vi "TwithFPO_DAQmx.vi"() -> ()   [LabVIEW 2019]
doc: "EE 200 Problem Set 7 Problem 25"
uses:
  Downloads/Project 2/Project 2/state.ctl
  <vilib>/DAQmx/read.llb/DAQmx Read (Digital 1D Bool 1Chan 1Samp).vi
  <vilib>/DAQmx/write.llb/DAQmx Write (Digital 1D Bool 1Chan 1Samp).vi
  <vilib>/DAQmx/write.llb/DAQmx Write (Analog DBL 1Chan 1Samp).vi
  <vilib>/DAQmx/read.llb/DAQmx Read (Digital Bool 1Line 1Point).vi
  <vilib>/DAQmx/create/channels.llb/DAQmx Create Channel (DI-Digital Input).vi
  <vilib>/DAQmx/create/channels.llb/DAQmx Create Channel (DO-Digital Output).vi
  <vilib>/DAQmx/create/channels.llb/DAQmx Create Channel (AO-Voltage-Basic).vi
  <vilib>/DAQmx/miscellaneous.llb/DAQmx Fill In Error Info.vi
panel:
  out "Thermostat Signal":u32[](array[colorbox])
  out "Reset":bool
  out "Clock":bool
  out "Present State":T1
  out "Clock Cycle":i32
  out "Sensors":bool[](array[boolean])
  in  "Stop Button":bool
  # "Thermostat"
  # "H\n\nC\n\nB"
  # "Standby \n\n\nCharging\n\n\nCooling\n\n\nHeating"
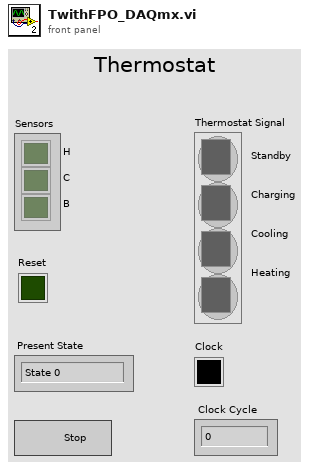
[diagram p1: front panel]
types:
  T1 = typedef "state.ctl" = enum16{"State 0", "State 1", "State 2", "State 3"}
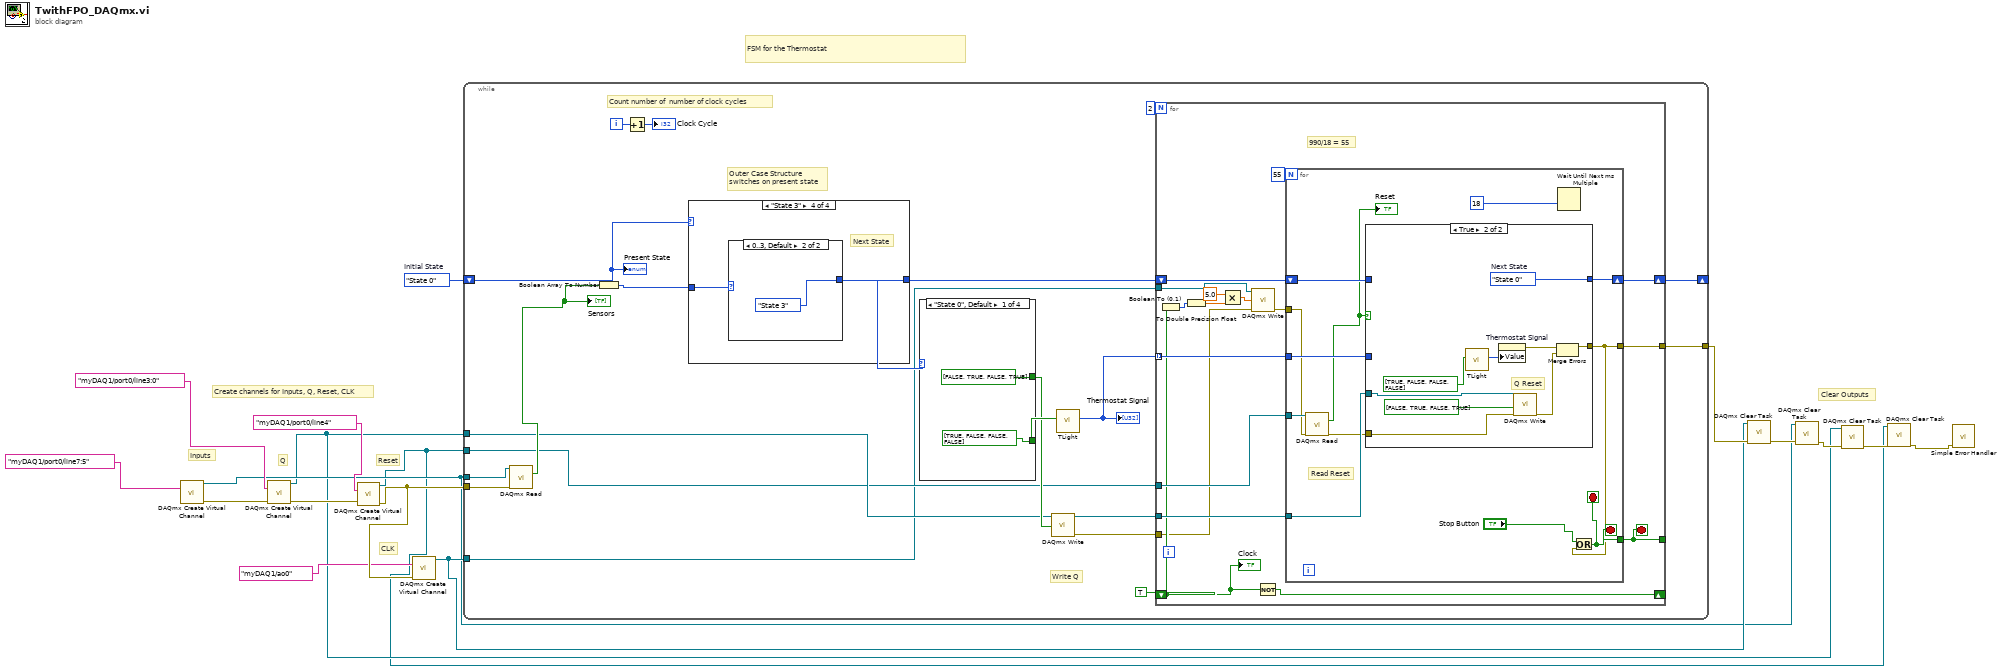
[diagram p0: block diagram]
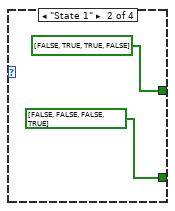
[diagram p2: hidden frame]
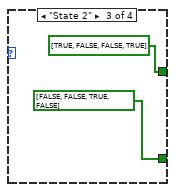
[diagram p3: hidden frame]
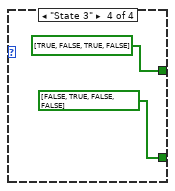
[diagram p4: hidden frame]
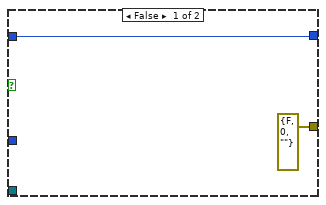
[diagram p5: hidden frame]
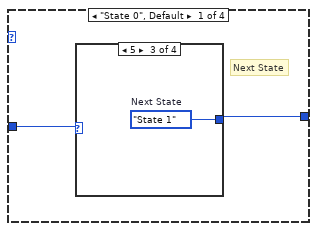
[diagram p6: hidden frame]
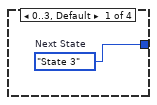
[diagram p7: hidden frame]
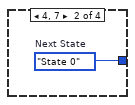
[diagram p8: hidden frame]
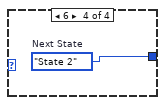
[diagram p9: hidden frame]
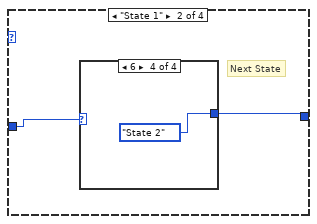
[diagram p10: hidden frame]
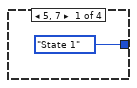
[diagram p11: hidden frame]
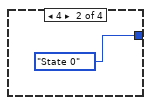
[diagram p12: hidden frame]
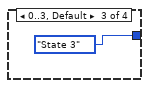
[diagram p13: hidden frame]
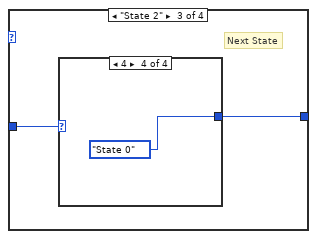
[diagram p14: hidden frame]
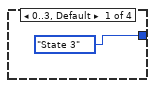
[diagram p15: hidden frame]
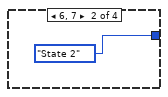
[diagram p16: hidden frame]
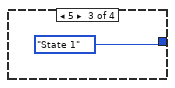
[diagram p17: hidden frame]
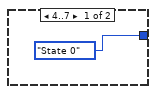
[diagram p18: hidden frame]
diagram:
  w17 = state."State 0"  # Initial State
  # "Clear Outputs"
  # "Create channels for Inputs, Q, Reset, CLK"
  # "CLK"
  # "Reset"
  # "Q"
  # "Inputs"
  # "FSM for the Thermostat"
  n1 = call-poly <vilib>:"DAQmx Create Virtual Channel.vi"("lines"=tag "myDAQ1/port0/line7:5") -> ("task out"=w3:refnum<k21>, "error out"=w16:errorcluster)  [unwired: 13 in]
  n2 = call-poly <vilib>:"DAQmx Create Virtual Channel.vi"("lines"=tag "myDAQ1/port0/line3:0", "error in"=w16) -> ("task out"=w2:refnum<k21>, "error out"=w15:errorcluster)  [unwired: 12 in]
  n3 = call-poly <vilib>:"DAQmx Create Virtual Channel.vi"("lines"=tag "myDAQ1/port0/line4", "error in"=w15) -> ("task out"=w1:refnum<k21>, "error out"=w14:errorcluster)  [unwired: 12 in]
  n4 = call-poly <vilib>:"DAQmx Create Virtual Channel.vi"("physical channels"=tag "myDAQ1/ao0", "error in"=w14) -> ("task out"=w8:refnum<k21>)  [unwired: 12 in, 1 out]
  n5 = while {
    shift-right: [w33] -> _
    shift-left: w17 -> [w36]
    tunnel: [w31] -> w9
    tunnel: w3 -> [w27]
    tunnel: w14 -> [w26]
    tunnel: w2 -> [w22]
    tunnel: w1 -> [w20]
    tunnel: w8 -> [w19]
    i -> [w38]
    stop <- w35 stop-if-true
    # "Write Q"
    # "Count number of  number of clock cycles"
    # "Outer Case Structure \nswitches on present state"
    n6 = call-poly <vilib>:"DAQmx Read.vi"("task/channels in"=w27, "error in"=w26) -> ("data"=w25:bool[])  [unwired: 11 in, 2 out]
    "Sensors" <- w25
    n7 = Boolean Array To Number(Boolean array=w25) -> (number=w28:u32)
    n8 = Increment(x=w38) -> (x+1=→"Clock Cycle":i32)
    n9 = case shown="\"State 3\"" w36 {
      tunnel: [w88 w94 w100 w106] -> w32
      tunnel: w28 -> [w87 w93 w99 w105]
      frame "State 0", Default {
        # "Next State"
        n10 = case shown="5" w87 {
          tunnel: [w89 w90 w91 w92] -> w88
          frame 0..3, Default {
            w89 = state."State 3"  # Next State
          }
          frame 4, 7 {
            w90 = state."State 0"  # Next State
          }
          frame 5 {
            w91 = state."State 1"  # Next State
          }
          frame 6 {
            w92 = state."State 2"  # Next State
          }
        }
      }
      frame "State 1" {
        # "Next State"
        n11 = case shown="6" w93 {
          tunnel: [state."State 1" ("Present State") state."State 0" ("Present State") state."State 3" ("Present State") state."State 2" ("Present State")] -> w94
          frame 5, 7 {
          }
          frame 4 {
          }
          frame 0..3, Default {
          }
          frame 6 {
          }
        }
      }
      frame "State 2" {
        # "Next State"
        n12 = case shown="4" w99 {
          tunnel: [state."State 3" ("Present State") state."State 2" ("Present State") state."State 1" ("Present State") state."State 0" ("Present State")] -> w100
          frame 0..3, Default {
          }
          frame 6, 7 {
          }
          frame 5 {
          }
          frame 4 {
          }
        }
      }
      frame "State 3" {
        # "Next State"
        n13 = case shown="0..3, Default" w105 {
          tunnel: [state."State 0" ("Present State") state."State 3" ("Present State")] -> w106
          frame 4..7 {
          }
          frame 0..3, Default {
          }
        }
      }
    }
    n14 = case shown="\"State 0\", Default" w32 {
      tunnel: [bool[] [TRUE, FALSE, FALSE, FALSE] bool[] [FALSE, FALSE, FALSE, TRUE] bool[] [FALSE, FALSE, TRUE, FALSE] bool[] [FALSE, TRUE, FALSE, FALSE]] -> w24
      tunnel: [bool[] [FALSE, TRUE, FALSE, TRUE] bool[] [FALSE, TRUE, TRUE, FALSE] bool[] [TRUE, FALSE, FALSE, TRUE] bool[] [TRUE, FALSE, TRUE, FALSE]] -> w23
      frame "State 0", Default {
      }
      frame "State 1" {
      }
      frame "State 2" {
      }
      frame "State 3" {
      }
    }
    n15 = call-poly <vilib>:"DAQmx Write.vi"("task/channels in"=w22, "data"=w23) -> ("task out"=w21:refnum<k21>, "error out"=w18:errorcluster)  [unwired: 11 in, 1 out]
    n16 = call "TLight.vi"("Array"=w24) -> ("Array 2"=w30:u32[])  [unwired: 10 in]
    "Thermostat Signal" <- w30
    n17 = for {
      N: 2 -> [_]
      shift-right: [w61] -> w33
      shift-left: w32 -> [w62]
      tunnel: [w63] -> w35
      shift-right: [w59] -> _
      shift-left: TRUE -> [w54]
      tunnel: [w60] -> w31
      tunnel: w30 -> [w58] mode=indexing
      tunnel: w21 -> [w56]
      tunnel: w20 -> [w55]
      tunnel: w19 -> [w49]
      tunnel: w18 -> [w48]
      stop <- w63 stop-if-true
      # "990/18 = 55"
      n18 = Boolean To (0,1)(Boolean=w54) -> (0, 1=w53:i16)
      n19 = To Double Precision Float(number=w53) -> (double precision float=w51:dbl)
      n20 = Multiply(x=5.0, y=w51) -> (x*y=w52:dbl)
      n21 = call-poly <vilib>:"DAQmx Write.vi"("task/channels in"=w49, "data"=w52, "error in"=w48) -> ("error out"=w47:errorcluster)  [unwired: 10 in, 2 out]
      n22 = Not(x=w54) -> (.not. x?=w59:bool)
      n23 = for {
        N: 55 -> [_]
        tunnel: [w64] -> w63
        shift-right: [w75] -> w61
        shift-left: w62 -> [w74]
        tunnel: [w65] -> w60
        tunnel: w58 -> [w73]
        tunnel: w56 -> [w72]
        tunnel: w55 -> [w70]
        tunnel: w47 -> [w68]
        stop <- w64 stop-if-true
        # "Read Reset"
        n24 = call-poly <vilib>:"DAQmx Read.vi"("task/channels in"=w70, "error in"=w68) -> ("data"=w71:bool, "error out"=w67:errorcluster)  [unwired: 11 in, 1 out]
        "Reset" <- w71
        n25 = case shown="True" w71 {
          tunnel: [w77 w86] -> w75
          tunnel: w74 -> [w77 _]
          tunnel: [errorcluster {"status"=FALSE, "code"=0, "source"=""} ("error constant") w85] -> w65
          tunnel: w73 -> [_ _]
          tunnel: w72 -> [_ w79]
          tunnel: w67 -> [_ w78]
          frame False {
          }
          frame True {
            w86 = state."State 0"  # Next State
            # "Q Reset"
            n26 = call "TLight.vi"("Array"=bool[] [TRUE, FALSE, FALSE, FALSE]) -> ("Array 2"=w82:u32[])  [unwired: 10 in]
            n27 = property on="Thermostat Signal" class="Arr (strict)"("Value"=w82) -> (error out=w84:errorcluster)  [unwired: 2 in, 1 out]
            n28 = call-poly <vilib>:"DAQmx Write.vi"("task/channels in"=w79, "data"=bool[] [FALSE, TRUE, FALSE, TRUE], "error in"=w78) -> ("error out"=w80:errorcluster)  [unwired: 10 in, 2 out]
            n29 = Merge Errors(w84, w80) -> (w85:errorcluster)
          }
        }
        n30 = Wait Until Next ms Multiple(millisecond multiple=u32 18 ("milliseconds to wait")) -> ()  [unwired: 1 out]
        n31 = Or(x="Stop Button", y=w65) -> (x .or. y?=w64:bool)
      }
      "Clock" <- w54
    }
    "Present State" <- w36
  }
  n32 = call <vilib>:"DAQmx Clear Task.vi"("task in"=w8, "error in"=w9) -> ("error out"=w7:errorcluster)  [unwired: 13 in]
  n33 = call <vilib>:"DAQmx Clear Task.vi"("task in"=w3, "error in"=w7) -> ("error out"=w6:errorcluster)  [unwired: 13 in]
  n34 = call <vilib>:"DAQmx Clear Task.vi"("task in"=w2, "error in"=w6) -> ("error out"=w5:errorcluster)  [unwired: 13 in]
  n35 = call <vilib>:"DAQmx Clear Task.vi"("task in"=w1, "error in"=w5) -> ("error out"=w4:errorcluster)  [unwired: 13 in]
  n36 = call <vilib>:"Simple Error Handler.vi"("error in (no error)"=w4) -> ()  [unwired: 4 in, 5 out]
